vi "Calculate_position.vi"(8 "P(theta)":dbl format="%#_13g", 11 "P0":dbl format="%#_13g") -> (3 "theta":dbl format="%#_13g")   [LabVIEW 2021]
doc: "This VI enables to calculate the rotation angle [°] required to move the filter to the specified position, for which the power level is equal to P(theta).\n\nInputs:\n(1) P0 - the power of the laser (for the position, for which the filter is transparent => T=100%)\n(2) P(theta) - the power level\n\nOutputs:\n(1) abs(theta) - the absolute value of the rotation angle in [°]\n(2) sign - the rotation angle sign (+1 or -1)"
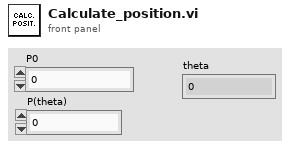
[diagram p1: front panel]
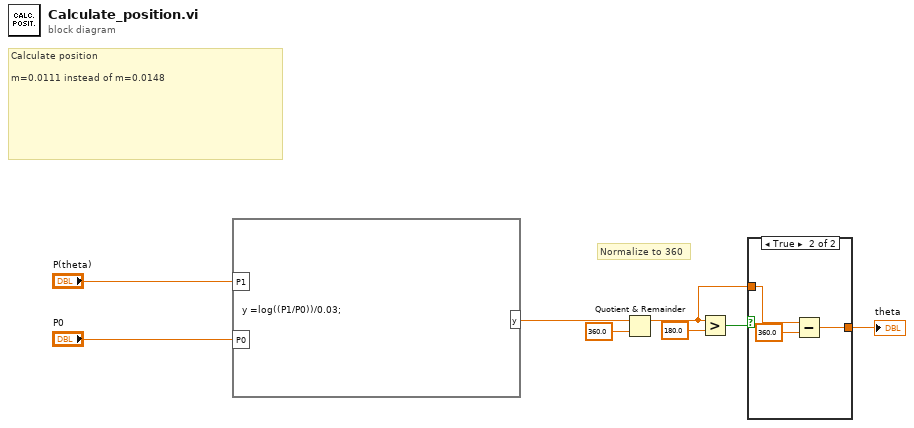
[diagram p0: block diagram]
diagram:
  # "Normalize to 360"
  # "Calculate position\n\nm=0.0111 instead of m=0.0148"
  n1 = formula code="y =log((P1/P0))/0.03;"("P0"="P0", "P1"="P(theta)") -> ("y"=w7:dbl)
  n2 = Quotient & Remainder(x=w7, y=360.0) -> (x-y*floor(x/y)=w3:dbl)  [unwired: 1 out]
  n3 = Greater?(x=w3, y=180.0) -> (0:w4:bool)
  n4 = case shown="True" w4 {
    tunnel: w3 -> [w9 w12]
    tunnel: [w9 w11] -> w1
    frame False {
    }
    frame True {
      n5 = Subtract(x=w12, y=360.0) -> (x-y=w11:dbl)
    }
  }
  "theta" <- w1
